vi "Get Image Flip.vi"(8 "error in (no error)":errorcluster, 10 "iVFlip":i32, 11 "iHFlip":i32) -> (0 "error out":errorcluster, 1 "function return":u32, 2 "iVFlip out":i32, 3 "iHFlip out":i32)   [LabVIEW 2014, in "atmcd32d.lvlib"]
doc: "unsigned int WINAPI GetImageFlip(int * iHFlip, int * iVFlip);"
uses:
  atmcd32d.lvlib
  atmcd32d.dll
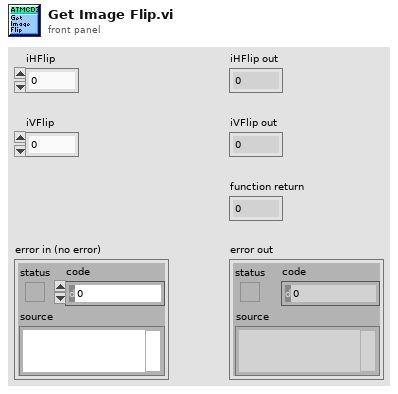
[diagram p1: front panel]
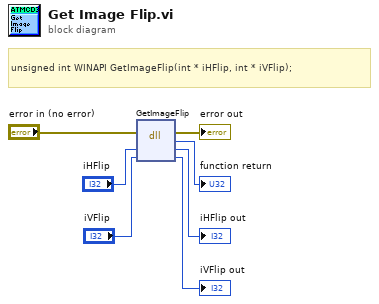
[diagram p0: block diagram]
diagram:
  # "unsigned int WINAPI GetImageFlip(int * iHFlip, int * iVFlip);"
  n1 = dll-call lib="C:/Users/Bakir/Documents/Lambda2-Testing/lib/Andorlib/atmcd32d.*" fn="GetImageFlip"(error in="error in (no error)", "iHFlip"="iHFlip", "iVFlip"="iVFlip") -> (error out=→"error out":errorcluster, →"function return":u32, "iHFlip"=→"iHFlip out":i32, "iVFlip"=→"iVFlip out":i32)  [unwired: 2 in, 1 out]
